vi "Network_Streams_Reader.vi"() -> ()   [LabVIEW 2014]
panel:
  out "error?":bool
  out "data out":string
  in  "stop":bool
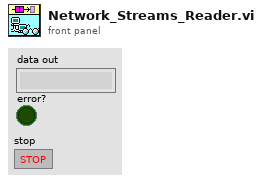
[diagram p1: front panel]
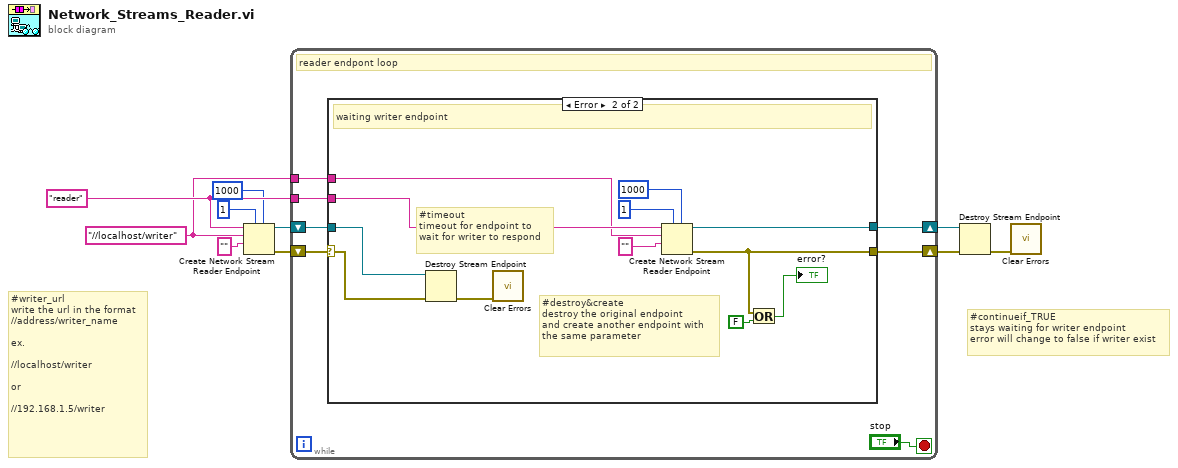
[diagram p0: block diagram]
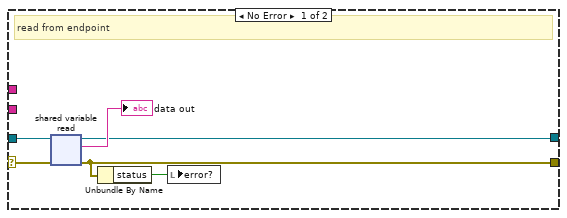
[diagram p2: hidden frame]
diagram:
  w3 = "//localhost/writer" ("writer url")
  w8 = "reader" ("reader name")
  # "#continueif_TRUE\nstays waiting for writer endpoint\nerror will change to false if writer exist"
  # "#writer_url\nwrite the url in the format\n//address/writer_name\n\nex.\n\n//localhost/writer\n\nor\n\n//192.168.1.5/writer"
  n1 = Create Network Stream Reader Endpoint(5:1000 ("timeout in ms (-1)"), 7:1 ("reader buffer size"), 9:"" ("writer url"), 10:w3, 11:w8) -> (0:w10:errorcluster, 3:w9:refnum<k21>)  [unwired: 2 in]
  n2 = while {
    tunnel: w8 -> [w14]
    shift-right: [w12] -> w5
    shift-left: w10 -> [w16]
    tunnel: w3 -> [w11]
    shift-right: [w13] -> w6
    shift-left: w9 -> [w15]
    stop <- "stop" stop-if-true
    # "reader endpont loop"
    n3 = case shown="Error" w16 {
      selector: w16 -> [w23 w35]
      tunnel: w15 -> [w22 w34]
      tunnel: w14 -> [_ w33]
      tunnel: [w20 w32] -> w13
      tunnel: [w19 w31] -> w12
      tunnel: w11 -> [_ w30]
      frame No Error {
        # "read from endpoint"
        n4 = shared-variable-read(w22, w23) -> (w20:refnum<k21>, w19:errorcluster, →"data out":string)  [unwired: 1 in, 1 out]
        n5 = Unbundle By Name(w19) -> ("status"=w18:bool)
        n6 = local write "error?"(w18) -> ()
      }
      frame Error {
        # "#timeout\ntimeout for endpoint to\nwait for writer to respond"
        # "#destroy&create\ndestroy the original endpoint\nand create another endpoint with\nthe same parameter"
        # "waiting writer endpoint"
        n7 = Destroy Stream Endpoint(8:w35, 11:w34) -> (0:w29:errorcluster)
        n8 = call <vilib>:"Clear Errors.vi"("error in (no error)"=w29) -> ()  [unwired: 5 in, 2 out]
        n9 = Create Network Stream Reader Endpoint(5:1000 ("reader buffer size"), 7:1 ("reader buffer size"), 9:"" ("writer url"), 10:w30, 11:w33) -> (0:w31:errorcluster, 3:w32:refnum<k21>)  [unwired: 2 in]
        n10 = Or(x=w31, y=FALSE) -> (x .or. y?=→"error?":bool)
      }
    }
  }
  n11 = Destroy Stream Endpoint(8:w5, 11:w6) -> (0:w2:errorcluster)
  n12 = call <vilib>:"Clear Errors.vi"("error in (no error)"=w2) -> ()  [unwired: 5 in, 2 out]
